vi "WS1050 16 DUT VSA-CV Sweep Ver1.1.vi"() -> ()   [LabVIEW 2012]
uses:
  Type Defs/WSVCAP SHL I2C DUT Mask Mode Enum.ctl
  <vilib>/Utility/file.llb/Read From Spreadsheet File (DBL).vi
  SubVI/Agilent E363X Series/Agilent E363X Series.lvlib
  SubVI/keithley_2000/Keithley 2000/Keithley 2000.lvlib
  SubVI/2012_Keithley 24XX/Keithley 24XX.lvlib
panel:
  out "Voltage Out":dbl[](array[numeric])
  out "C1 Out":dbl[][](array[numeric])
  out "VISA resource name out":refnum<visa-resource-name>="GPIB0::3::INSTR"
  out "date string":string="5/19/2014"
  out "PS1 Out":refnum<visa-resource-name>
  out "Ke2000 Out":refnum<visa-resource-name>="GPIB0::9::INSTR"
  in  "Tab Control":enum32{"Inst Control", "Data Output", "Graphs"}(tab)=enum."Data Output"
  out "AD7747 Values":string[][](table)
  in  "Lot#":string="WS1050"
  in  "Wafer#":string="T7-EB"
  in  "File Name":string="WS1050_T7_VSA_CV"
  in  "TMN DC\\CAP Data Log File Path":path=path "C:/WS1050 16 DUT Data"
  in  "SN":string[](array[string])=["1", "2", "3", "4", "5", "6", "7", "8", "9", "10", "11", "12", "13", "14", "15", "16"]
  in  "Test Program":string="WS1050 16 DUT VSA_CV Sweep Ver1.0"
  out "Current Date":string="8/28/2014"
  out "Current Time":string="0950"
  in  "Start Date":string="4/24/2014"
  in  "Start Time":string="1542"
  in  "Comment":string="5X0p5"
  in  "OK Button":bool
  in  "Calibration":bool
  in  "Control Setting":bool
  in  "CP Setting":i32(ring) items=["CP OFF", "CP ON", "CP 35V", "CP 40V", "DVA OFF", "DVA ON", "Reg1 ON", "Reg1 OFF", "Reg2 ON", "Reg2 OFF", "Reg3 ON", "Reg3 OFF"]
  in  "VDD(V)":dbl=3.3 format="%.3g"
  in  "SPI Clock Rate (Hz)":dbl=1000000.0 caption="Meas Speed" format="%.1p Hz"
  out "AR  Measurent(Hz)":dbl
  in  "PS1 Source":refnum<visa-resource-name>="GPIB0::5::INSTR"
  in  "Ke2000":refnum<visa-resource-name>="GPIB0::9::INSTR"
  out "Simulate FPGA":bool
  out "Online":bool
  in  "Ke2400":refnum<visa-resource-name>="GPIB0::3::INSTR"
  in  "Initialize AD7747":bool
  in  "DUT Mask Mode":T1=enum."All"
  in  "RFFE Slave Address":u8=7 caption="Slave Address" format="0x%02x"
  out "Activity Log":string="05/19/2014 -- 12:24:35.853::WSVCAP::APP::Application Started\n05/19/2014 -- 12:24:37.606::WSVCAP::WSVCAP SHL::WR I2C-REG:0x0A;MASK:0xFFFFFFFFFFFF;C1 DATA:22:22:22:22:22:22:22:22:22:22:22:22:22:22:22:22;C2 DATA:22:22:22:22:22:22:22:22:22:22:22:22:22:22:22:22;C3 DATA:22:22:22:22:22:22:22:22:22:22:22:22:22:22:22:22\r\n05/19/2014 -- 12:24:37.773::WSVCAP::WSVCAP SHL::WR I2C-ST:0,0,4,1\r\n05/19/2014 -- 12:24:37.903::WSVCAP::WSVCAP SHL::RD I2C-BYTES:4;ADD:0x00;MASK:0xFFFFFFFFFFFF\r\n05/19/2014 -- 12:24:38.045::WSVCAP::WSVCAP SHL::RD I2C:C1 DATA:2:2:2:2:2:2:2:2:2:2:2:2:2:2:2:2|A7:A9:AA:82:82:7F:82:81:82:81:83:82:81:82:82:81|46:36:BB:88:44:A3:E9:2B:32:20:ED:25:BB:3D:68:B|2C:6A:EB:A7:22:56:FE:CC:36:82:D7:B0:3B:48:F9:CC;C2 DATA:2:2:2:2:2:2:2:2:2:2:2:2:2:2:2:2|94:94:94:80:80:80:80:80:81:7E:7E:81:80:7E:80:80|47:33:15:82:62:B:E8:1C:D7:C3:7D:41:7C:B7:4C:2A|C4:B4:AE:8:1E:D1:4E:37:11:C0:6F:63:42:9D:63:B5;C3 DATA:2:2:2:2:2:2:2:2:2:2:2:2:2:2:2:2|95:95:95:81:81:7E:81:80:84:7D:80:83:81:7E:7F:80|AB:C4:14:B5:7B:52:DF:C9:79:5D:5F:30:99:31:1E:F4|6E:5C:F7:A8:C3:EB:7B:EF:33:92:89:77:4D:67:75:DD;STATUS:0:0:4:0\r\n05/19/2014 -- 12:24:38.046::WSVCAP::WSVCAP SHL::WR I2C-REG:0x0A;MASK:0xFFFFFFFFFFFF;C1 DATA:22:22:22:22:22:22:22:22:22:22:22:22:22:22:22:22;C2 DATA:22:22:22:22:22:22:22:22:22:22:22:22:22:22:22:22;C3 DATA:22:22:22:22:22:22:22:22:22:22:22:22:22:22:22:22\r\n05/19/2014 -- 12:24:38.089::WSVCAP::WSVCAP SHL::WR I2C-ST:0,0,4,1\r\n05/19/2014 -- 12:24:38.219::WSVCAP::WSVCAP SHL::RD I2C-BYTES:4;ADD:0x00;MASK:0xFFFFFFFFFFFF\r\n05/19/2014 -- 12:24:38.362::WSVCAP::WSVCAP SHL::RD I2C:C1 DATA:2:2:2:2:2:2:2:2:2:2:2:2:2:2:2:2|A7:AB:AA:82:82:82:83:83:82:82:82:82:7F:82:82:81|4B:32:96:83:3E:61:43:17:25:62:AB:4D:A2:40:2E:5|3C:76:2B:B4:EE:E4:A9:1A:AA:A:26:C7:21:2E:87:5B;C2 DATA:2:2:2:2:2:2:2:2:2:2:2:2:2:2:2:2|94:94:94:80:80:80:80:80:80:7F:80:81:80:80:7F:80|4A:32:19:7D:19:6C:79:46:61:7F:4B:B8:A5:30:F3:14|B4:70:A:8C:9C:DC:43:FA:1E:A:C6:21:A:A9:13:F3;C3 DATA:2:2:2:2:2:2:2:2:2:2:2:2:2:2:2:2|95:97:94:81:80:81:82:81:80:7E:81:84:7F:81:80:80|B2:32:D0:A7:9E:4C:AB:D4:EE:D9:F0:82:B7:91:7:FF|C1:91:B6:3D:D8:E:1B:4F:9F:6A:F1:6C:E7:3F:7:BA;STATUS:0:0:4:0\r\n05/19/2014 -- 12:24:38.364::WSVCAP::WSVCAP SHL::WR I2C-REG:0x0A;MASK:0xFFFFFFFFFFFF;C1 DATA:22:22:22:22:22:22:22:22:22:22:22:22:22:22:22:22;C2 DATA:22:22:22:22:22:22:22:22:22:22:22:22:22:22:22:22;C3 DATA:22:22:22:22:22:22:22:22:22:22:22:22:22:22:22:22\r\n05/19/2014 -- 12:24:38.406::WSVCAP::WSVCAP SHL::WR I2C-ST:0,0,4,1\r\n05/19/2014 -- 12:24:38.536::WSVCAP::WSVCAP SHL::RD I2C-BYTES:4;ADD:0x00;MASK:0xFFFFFFFFFFFF\r\n05/19/2014 -- 12:24:38.678::WSVCAP::WSVCAP SHL::RD I2C:C1 DATA:2:2:2:2:2:2:2:2:2:2:2:2:2:2:2:2|A7:A9:AB:82:82:81:82:82:82:82:82:82:82:82:82:81|46:71:4C:87:43:3D:7F:FC:25:4F:8E:54:97:3E:60:8C|AA:F4:1F:B5:CE:43:1F:36:9:87:9C:78:86:5:B6:8E;C2 DATA:2:2:2:2:2:2:2:2:2:2:2:2:2:2:2:2|94:94:94:80:7F:7F:80:80:80:80:80:81:80:80:80:80|49:36:18:7D:6E:C5:E4:3C:81:2E:41:D3:75:71:E3:72|E8:D3:E6:D1:E0:48:AE:D4:54:D:E8:8E:B4:41:68:4;C3 DATA:2:2:2:2:2:2:2:2:2:2:2:2:2:2:2:2|95:95:95:81:7F:7F:81:81:81:81:81:84:81:81:82:81|B3:F5:90:AB:82:69:7B:93:D0:77:E8:D5:E8:8C:84:E8|B9:AC:EE:2B:B6:71:8F:4A:74:31:56:BB:8A:B7:A0:C8;STATUS:0:0:4:0\r\n05/19/2014 -- 12:24:38.681::WSVCAP::WSVCAP SHL::WR I2C-REG:0x0A;MASK:0xFFFFFFFFFFFF;C1 DATA:22:22:22:22:22:22:22:22:22:22:22:22:22:22:22:22;C2 DATA:22:22:22:22:22:22:22:22:22:22:22:22:22:22:22:22;C3 DATA:22:22:22:22:22:22:22:22:22:22:22:22:22:22:22:22\r\n05/19/2014 -- 12:24:38.723::WSVCAP::WSVCAP SHL::WR I2C-ST:0,0,4,1\r\n05/19/2014 -- 12:24:38.854::WSVCAP::WSVCAP SHL::RD I2C-BYTES:4;ADD:0x00;MASK:0xFFFFFFFFFFFF\r\n05/19/2014 -- 12:24:38.996::WSVCAP::WSVCAP SHL::RD I2C:C1 DATA:2:2:2:2:2:2:2:2:2:2:2:2:2:2:2:2|A7:A9:AA:82:82:7F:83:81:82:81:84:82:7F:82:7F:82|43:FB:E:7F:3C:AD:35:35:26:A2:6C:21:4B:3D:8:6|63:9A:E1:F3:95:32:91:42:90:3C:78:1F:5C:D7:5F:D8;C2 DATA:2:2:2:2:2:2:2:2:2:2:2:2:2:2:2:2|94:94:94:80:80:80:80:80:81:80:7E:81:80:7E:7F:80|48:36:18:7F:5E:3D:69:83:DE:AE:A1:9E:31:AE:BB:96|15:A0:44:17:13:FD:CC:C8:6D:B2:EF:A7:C:C7:3B:F;C3 DATA:2:2:2:2:2:2:2:2:2:2:2:2:2:2:2:2|95:96:94:81:81:7E:82:80:84:80:80:84:7F:7E:7D:82|AD:3B:6D:A9:7C:57:9D:F5:7A:96:23:5C:36:2D:ED:5A|CD:46:DB:3B:C7:BD:70:60:33:B8:B:F7:63:A:51:4D;STATUS:0:0:4:0\r\n05/19/2014 -- 12:24:38.998::WSVCAP::WSVCAP SHL::WR I2C-REG:0x0A;MASK:0xFFFFFFFFFFFF;C1 DATA:22:22:22:22:22:22:22:22:22:22:22:22:22:22:22:22;C2 DATA:22:22:22:22:22:22:22:22:22:22:22:22:22:22:22:22;C3 DATA:22:22:22:22:22:22:22:22:22:22:22:22:22:22:22:22\r\n05/19/2014 -- 12:24:39.040::WSVCAP::WSVCAP SHL::WR I2C-ST:0,0,4,1\r\n05/19/2014 -- 12:24:39.170::WSVCAP::WSVCAP SHL::RD I2C-BYTES:4;ADD:0x00;MASK:0xFFFFFFFFFFFF\r\n05/19/2014 -- 12:24:39.311::WSVCAP::WSVCAP SHL::RD I2C:C1 DATA:2:2:2:2:2:2:2:2:2:2:2:2:2:2:2:2|A7:AA:AB:82:82:81:82:81:82:81:82:82:82:82:7F:82|44:F1:90:87:45:44:C8:2C:2C:F1:FC:1B:94:3B:3C:75|4A:49:95:19:99:73:64:3:23:24:F3:A2:5E:7F:C4:B6;C2 DATA:2:2:2:2:2:2:2:2:2:2:2:2:2:2:2:2|94:94:94:80:80:80:80:7F:80:80:7E:80:80:7E:7F:80|4C:36:17:7D:A8:9F:DE:C7:53:6D:8A:F4:41:A5:C6:E0|90:2E:24:C:D9:22:E4:76:3B:40:1D:53:33:B1:3E:4D;C3 DATA:2:2:2:2:2:2:2:2:2:2:2:2:2:2:2:2|95:97:95:81:81:7F:81:80:80:81:7F:82:81:7E:7D:82|AE:2B:A7:AB:CC:CD:A4:38:FD:17:80:F2:92:2D:45:C4|76:E5:D:B9:AD:B5:BA:8D:28:32:9E:42:B7:20:4A:D9;STATUS:0:0:4:0\r\n05/19/2014 -- 12:24:39.313::WSVCAP::WSVCAP SHL::WR I2C-REG:0x0A;MASK:0xFFFFFFFFFFFF;C1 DATA:22:22:22:22:22:22:22:22:22:22:22:22:22:22:22:22;C2 DATA:22:22:22:22:22:22:22:22:22:22:22:22:22:22:22:22;C3 DATA:22:22:22:22:22:22:22:22:22:22:22:22:22:22:22:22\r\n05/19/2014 -- 12:24:39.355::WSVCAP::WSVCAP SHL::WR I2C-ST:0,0,4,1\r\n05/19/2014 -- 12:24:39.486::WSVCAP::WSVCAP SHL::RD I2C-BYTES:4;ADD:0x00;MASK:0xFFFFFFFFFFFF\r\n05/19/2014 -- 12:24:39.628::WSVCAP::WSVCAP SHL::RD I2C:C1 DATA:2:2:2:2:2:2:2:2:2:2:2:2:2:2:2:2|A7:A9:AA:82:82:82:83:82:82:82:82:82:7F:82:7F:82|47:18:E4:87:3E:E7:6:65:25:92:37:38:A8:3E:89:85|7C:A7:7:2B:A3:7A:EC:EF:89:ED:F4:D3:D8:BC:3A:F5;C2 DATA:2:2:2:2:2:2:2:2:2:2:2:2:2:2:2:2|94:94:94:80:7F:80:80:7F:81:80:7E:80:80:80:81:80|49:37:17:80:76:25:6A:F8:DF:55:97:4D:B8:5B:2B:B1|13:E3:9A:3E:1A:2D:4F:B6:DB:E9:61:FA:8B:D6:9:CC;C3 DATA:2:2:2:2:2:2:2:2:2:2:2:2:2:2:2:2|95:95:95:81:7F:80:82:81:84:80:7F:81:80:81:7F:82|AF:93:3B:AF:5B:11:82:E4:7E:C3:2D:72:9:96:D9:A|DB:96:F2:10:5F:64:9A:C6:98:12:27:7D:10:D3:20:D9;STATUS:0:0:4:0\r\n05/19/2014 -- 12:24:40.132::WSVCAP::WSVCAP SHL::CLOSE\r\n"
  in  "C1 Cap DAC":u8=128 caption="B Data In" format="0x%02x"
  in  "C2 Cap DAC":u8=128 caption="B Data In" format="0x%02x"
  in  "C3 Cap DAC":u8=128 caption="B Data In" format="0x%02x"
  out "IDD Brd(uA)":string
  in  "VSA_IDD(A)":dbl=0.1
  out "Previous Time":string="12:20:26 PM"
  out "STATUS":string="Idle...."
  in  "stop":bool
  out "VSA_C1_T0":string[](array[string])
  out "VSA_Value(pF)":string[][](array[string])
  out "VSA_C3_T0":string[](array[string])
  out "VSA_C2_T0":string[](array[string])
  in  "VSA Voltag Path":path=path "C:/VSA Voltage Sweep/VSA_Voltage_Seq_0-10-24V Step2V.txt"
  in  "VSA_CV Voltage Path":path=path "C:/VSA Voltage Sweep/VSA_Voltage_Seq_0-10-24V Step2V.txt"
  out "CP Current(uA)":string[](array[string])
  in  "Abort":bool
  out "Running Loops":i32=1
  in  "VSA_CV Reg Setting":i32(ring) items=["Reg1 ON", "Reg1 OFF", "Reg2 ON", "Reg2 OFF", "Reg3 ON", "Reg3 OFF", "All ON", "All OFF"]
  in  "VSA Test":bool=TRUE
  in  "error in (no error)":errorcluster
  out "error out":errorcluster
  out "error out 2":errorcluster
  out "Bank 3 Graph":cluster{"Y":dbl[], "Y":dbl[]}[](graph)
  out "Bank 2 Graph":cluster{"Y":dbl[], "Y":dbl[]}[](graph)
  out "Bank 1 Graph":cluster{"Y":dbl[], "Y":dbl[]}[](graph)
  out "C2 Plot":dbl[][](graph)
  out "C1 Plot":dbl[][](graph)
  out "C3 Plot":dbl[][](graph)
  # "Company:  WiSpry Inc 20 Fairbanks \nSte 198 Irvine CA 92618\n\nAuthor:  Andy V Tran\nCreated:  09/16/2015\nLabVIEW 2012 Pro\nTP:  WS1050 16 DUT VSA_CV Ver1.1\nFPGA Version: WS_VCAP Driver 024"
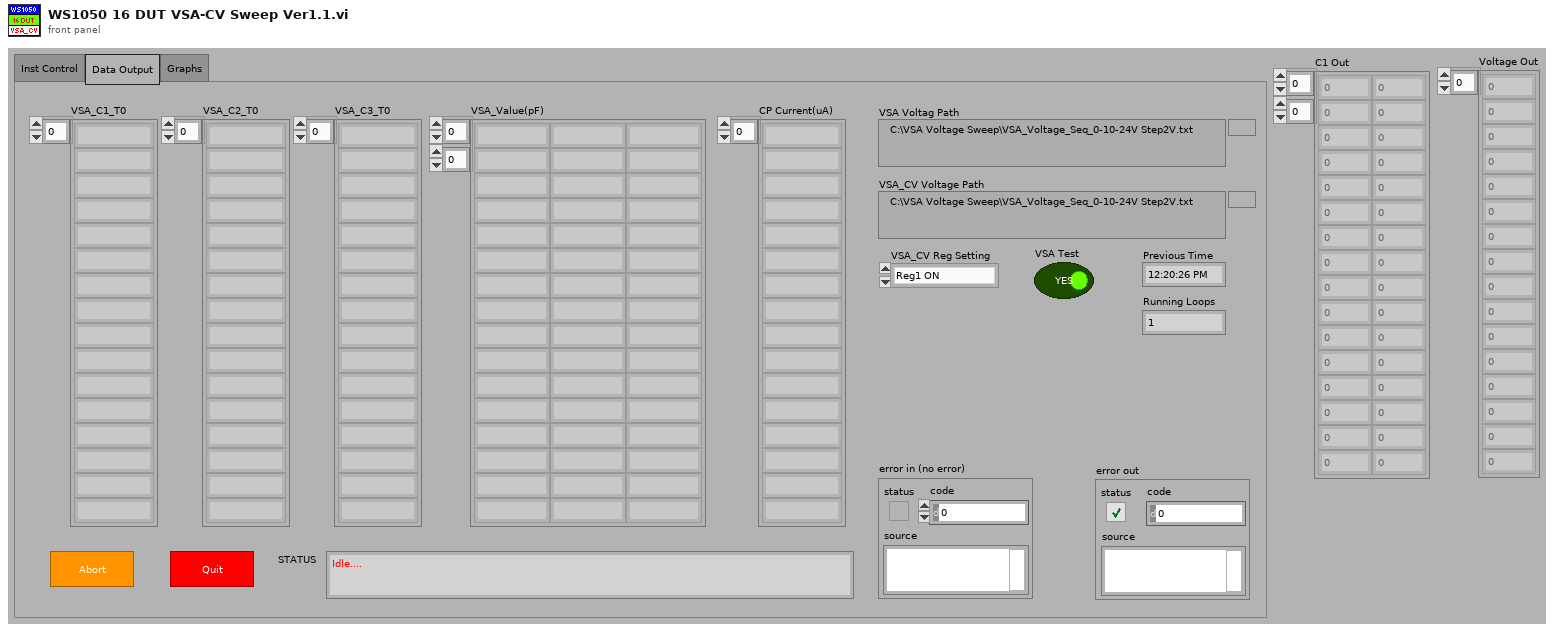
[diagram p1: front panel]
types:
  T1 = typedef "WSVCAP SHL I2C DUT Mask Mode Enum.ctl" = enum16{"Custom", "C1", "C2", "C3", "All"}
  T2 = typedef "WSVCAP SHL Core System Cluster.ctl" = cluster{"Settings":T3, "FPGA Resource":tag, "Online":bool, "I2C Wait Ticks":u32, "SPI Wait Ticks":u32, "RFFE Wait Ticks":u32}
  T3 = typedef "WSVCAP SHL I2C Settings Cluster.ctl" = cluster{"FPGA Resource Name":string, "I2C Slave Address":u8, "I2C Clock Rate (Hz)":dbl, "SPI Clock Rate (Hz)":dbl, "RFFE Slave Address":u8, "RFFE Clock Rate (Hz)":dbl, "Simulate FPGA":bool, "C1 Cap DAC Default":u8, "C2 Cap DAC Default":u8, "C3 Cap DAC Default":u8}
  T4 = enum16{"Idle...", "Voltage 1", "Voltage 2", "Voltage 3"}[]
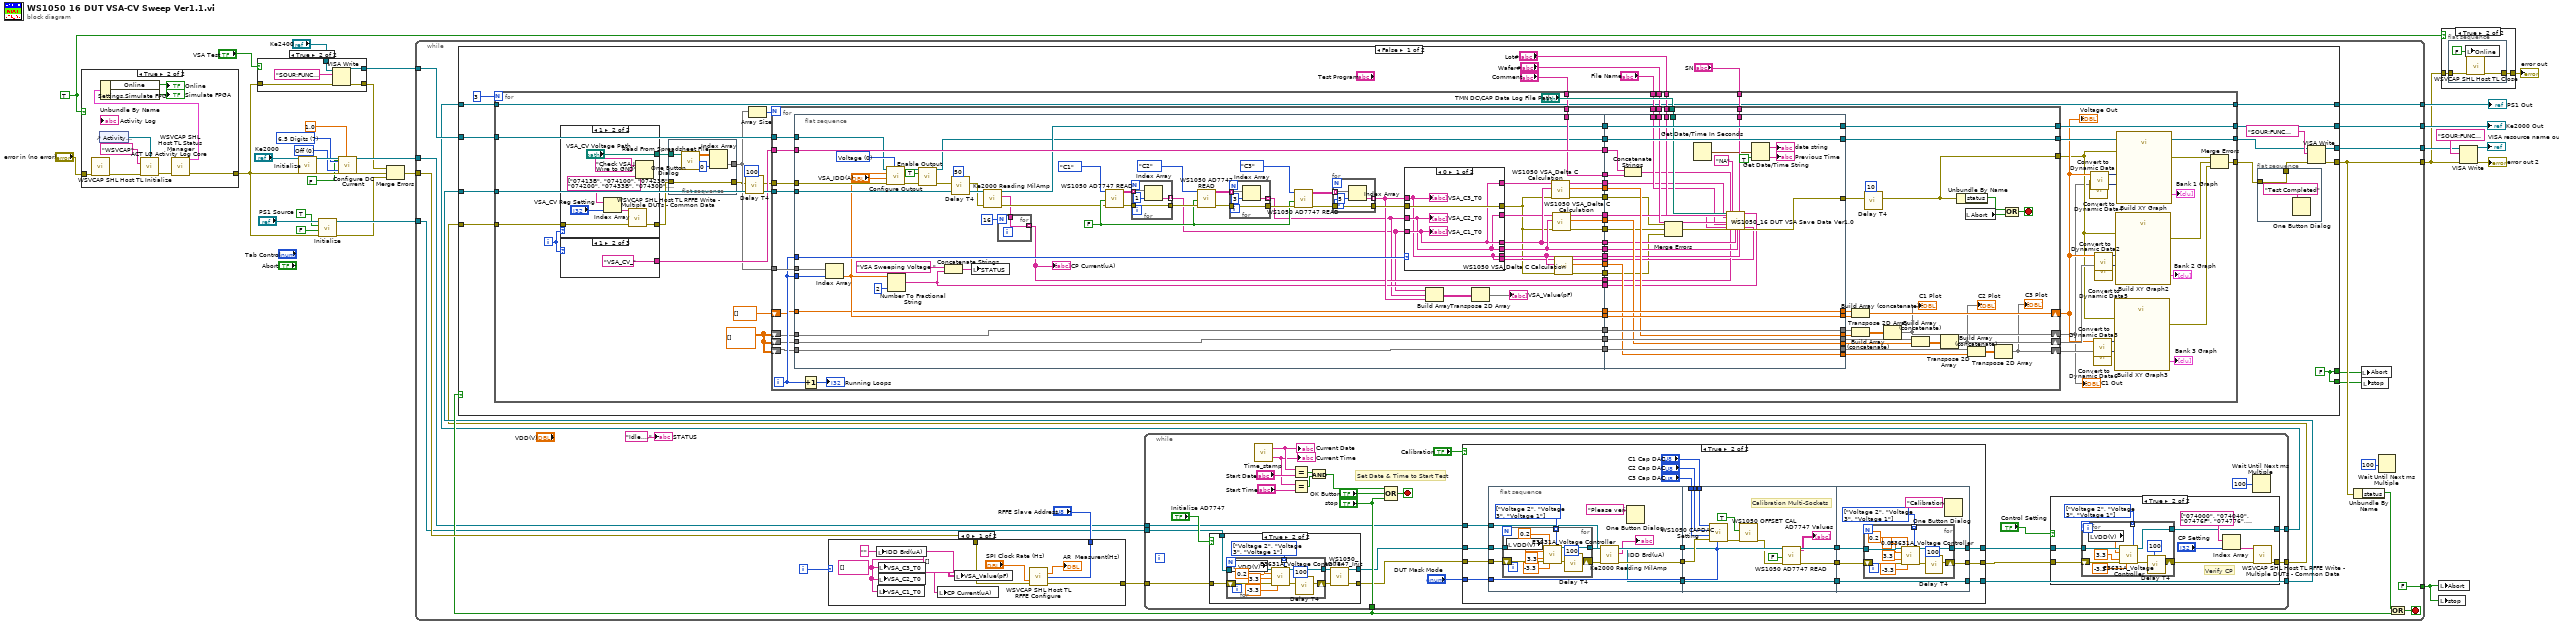
[diagram p0: block diagram]
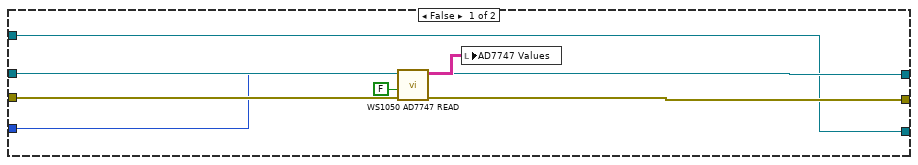
[diagram p8: hidden frame]
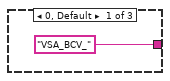
[diagram p9: hidden frame]
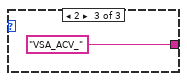
[diagram p10: hidden frame]
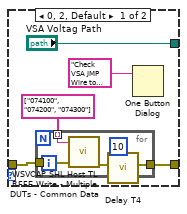
[diagram p11: hidden frame]
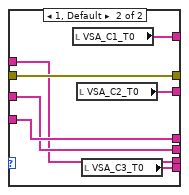
[diagram p12: hidden frame]
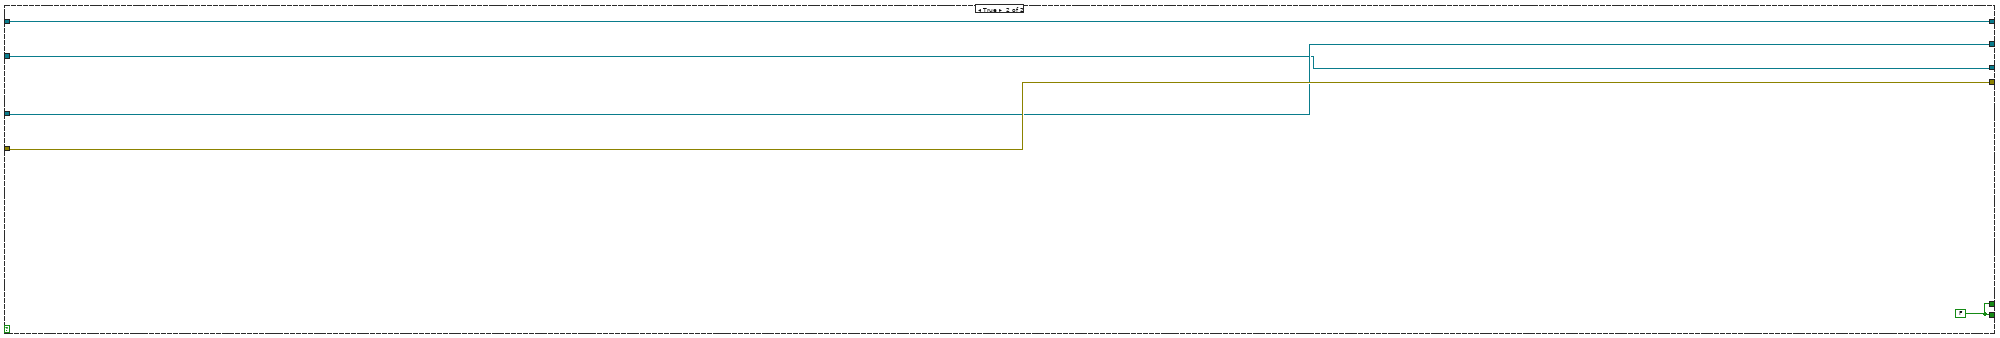
[diagram p13: hidden frame]
diagram:
  w17 = TRUE
  w23 = u16 0 items=["Off", "Moving Filter", "Repeating Filter"] ("Digital Filter (0: Off)")
  w24 = u16 7 items=["3.5 Digits"=4, "4.5 Digits"=5, "5.5 Digits"=6, "6.5 Digits"=7] ("Resolution (7: 6.5 digits)")
  n1 = case shown="True" w17 {
    tunnel: "error in (no error)" -> [w32 w33]
    tunnel: [w32 w40] -> w5
    frame False {
    }
    frame True {
      n2 = call "WSVCAP SHL Host TL Initialize.vi"("error in"=w33) -> ("error out"=w34:errorcluster)  [unwired: 13 in, 1 out]
      n3 = control-ref of="Activity Log"() -> (w36:refnum<vi>)
      n4 = call "ACT LG Activity Log Core.vi"("Display Ref"=w36, "Source"="WSVCAP", "Error In (no error)"=w34) -> ("Error Out"=w35:errorcluster)  [unwired: 11 in, 1 out]
      n5 = call "WSVCAP SHL Host TL Status Manager.vi"("error in"=w35) -> ("System Out"=w41:T2, "error out"=w40:errorcluster)  [unwired: 13 in]
      n6 = Unbundle By Name(w41) -> ("Online"=→"Online":bool, "Settings.Simulate FPGA"=→"Simulate FPGA":bool)
    }
  }
  n7 = case shown="True" "VSA Test" {
    tunnel: w5 -> [w42 w47]
    tunnel: [w43 w46] -> w14
    tunnel: [w42 w45] -> w9
    tunnel: "Ke2400" -> [w43 w44]
    frame False {
    }
    frame True {
      n8 = VISA Write(VISA resource name=w44, write buffer="SOUR:FUNC VOLT;VOLT:MODE FIX;RANG 100;LEV 0.0;:SENS:FUNC \"CURR\";CURR:PROT 60E-3;RANG 100E-3;:OUTP ON", error in (no error)=w47) -> (VISA resource name out=w46:refnum<visa-resource-name>, error out=w45:errorcluster)  [unwired: 1 out]
    }
  }
  n9 = call "Initialize.vi"("VISA resource name"="Ke2000", "error in (no error)"=w5) -> ("VISA resource name out"=w26:refnum<visa-resource-name>, "error out"=w25:errorcluster)  [unwired: 16 in]
  n10 = call "Initialize.vi"("error in (no error)"=w5, "Reset? (T: Yes)"=FALSE, "ID Query? (T: Yes)"=TRUE, "VISA resource name"="PS1 Source") -> ("error out"=w4:errorcluster, "VISA resource name out"=w29:refnum<visa-resource-name>)  [unwired: 6 in]
  n11 = call "Configure DC Current.vi"("VISA resource name"=w26, "Resolution (7: 6.5 digits)"=w24, "error in (no error)"=w25, "Auto Range? (T: Auto)"=FALSE, "Digital Filter (0: Off)"=w23, "Custom Range (0 A)"=1.0) -> ("VISA resource name out"=w21:refnum<visa-resource-name>, "error out"=w6:errorcluster)  [unwired: 12 in]
  n12 = Merge Errors(w9, w6, w4) -> (w15:errorcluster)
  n13 = while {
    tunnel: w15 -> [w63]
    tunnel: [w52] -> w11
    tunnel: w29 -> [w56]
    tunnel: w21 -> [w57]
    tunnel: [w66] -> w20
    tunnel: [w65] -> w19
    tunnel: w14 -> [w62]
    tunnel: [w61] -> w12
    tunnel: [FALSE] -> w3
    i -> [w64]
    stop <- w68 stop-if-true
    n14 = case shown="0" w64 {
      tunnel: w63 -> [w78 w79]
      tunnel: [w77 w79] -> w59
      tunnel: "RFFE Slave Address" -> [w75 _]
      frame 0 {
        w72 = string[] []
        n15 = local write "IDD Brd(uA)"("" ("uA")) -> ()
        n16 = local write "VSA_C1_T0"(w72) -> ()
        n17 = local write "VSA_C3_T0"(w72) -> ()
        n18 = local write "VSA_C2_T0"(w72) -> ()
        n19 = local write "CP Current(uA)"(w72) -> ()
        n20 = local write "VSA_Value(pF)"(string[][] []) -> ()
        n21 = call "WSVCAP SHL Host TL RFFE Configure.vi"("RFFE Slave Address"=w75, "Clock Rate (Hz)"="SPI Clock Rate (Hz)", "error in"=w78) -> ("Actual Rate (Hz)"=→"AR  Measurent(Hz)":dbl, "error out"=w77:errorcluster)  [unwired: 11 in]
      }
      frame 1, Default {
      }
    }
    n22 = while {
      tunnel: ["stop"] -> w60
      tunnel: w59 -> [w90]
      tunnel: [w81] -> w53
      tunnel: w56 -> [w88]
      tunnel: w57 -> [w83]
      tunnel: [w84] -> w55
      tunnel: [w82] -> w54
      stop <- w97 stop-if-true
      # "Set Date & Time to Start Test"
      n23 = case shown="True" "Initialize AD7747" {
        tunnel: w90 -> [w106 w111]
        tunnel: [w106 w107] -> w89
        tunnel: w88 -> [w105 w109]
        tunnel: [w105 w108] -> w87
        frame False {
        }
        frame True {
          w112 = T4 [enum."Voltage 2", enum."Voltage 3", enum."Voltage 1"] items=["Idle...", "Voltage 1", "Voltage 2", "Voltage 3"]
          n24 = for {
            tunnel: w109 -> [w122]
            tunnel: w112 -> [w119] mode=indexing
            tunnel: [w118] -> w108
            shift-right: [w114] -> w110
            shift-left: w111 -> [w123]
            n25 = local read "VDD(V)"() -> (w117:dbl)
            n26 = call "E3631A_Voltage Controller.vi"("VISA resource name"=w122, "I_VDD(A)"=0.2, "Channel Controller"=w119, "Voltage 1"=w117, "Voltage 2"=3.3, "error in (no error)"=w123, "Voltage 3"=-3.3) -> ("VISA resource name out"=w118:refnum<visa-resource-name>, "error out"=w113:errorcluster)  [unwired: 7 in]
            n27 = call "Delay T4.vi"("milliseconds to wait"=u32 100, "error in (no error)"=w113) -> ("error out"=w114:errorcluster)  [unwired: 9 in]
          }
          n28 = call "WS1050_AD7747_Init.vi"("error in"=w110) -> ("error out"=w107:errorcluster)  [unwired: 10 in]
        }
      }
      n29 = call "Time_stamp.vi"() -> ("date/time string"=w102:string, "date string"=w104:string)  [unwired: 2 in]
      "Current Date" <- w104
      "Current Time" <- w102
      n30 = Equal?(x=w104, y="Start Date") -> (x = y?=w100:bool)
      n31 = Equal?(x=w102, y="Start Time") -> (x = y?=w99:bool)
      n32 = And(x=w100, y=w99) -> (x .and. y?=w96:bool)
      n33 = Compound Arithmetic op=OR(w96, "OK Button", "stop") -> (w97:bool)
      n34 = case shown="True" "Calibration" {
        tunnel: w89 -> [w150 w168]
        tunnel: [w149 w165] -> w80
        tunnel: w87 -> [w148 w164]
        tunnel: "DUT Mask Mode" -> [w147 w160]
        tunnel: [w148 w159] -> w85
        tunnel: w83 -> [w146 w155]
        tunnel: [w146 w152] -> w82
        frame False {
          n35 = call "WS1050 AD7747 READ.vi"("error in"=w150, "Log (T)"=FALSE, "DUT Mask Mode (All)"=w147) -> ("error out"=w149:errorcluster, "AD7747 Values"=w151:string[][])  [unwired: 7 in]
          n36 = local write "AD7747 Values"(w151) -> ()
        }
        frame True {
          n37 = flat-sequence {
            tunnel: w168 -> [w177]
            tunnel: [w172] -> w167
            tunnel: w164 -> [w176]
            tunnel: [w175] -> w163
            tunnel: w160 -> [w174]
            tunnel: [w174] -> w161
            tunnel: w155 -> [w170]
            tunnel: [w169] -> w154
            tunnel: w167 -> [w203]
            tunnel: [w202] -> w166
            tunnel: w163 -> [w201]
            tunnel: [w201] -> w162
            tunnel: w161 -> [w200]
            tunnel: "C1 Cap DAC" -> [w196]
            tunnel: "C2 Cap DAC" -> [w195]
            tunnel: "C3 Cap DAC" -> [w194]
            tunnel: w154 -> [w193]
            tunnel: [w193] -> w153
            tunnel: w166 -> [w206]
            tunnel: [w209] -> w165
            tunnel: w162 -> [w208]
            tunnel: [w205] -> w159
            tunnel: w153 -> [w204]
            tunnel: [w204] -> w152
            frame #0 {
              w178 = T4 [enum."Voltage 2", enum."Voltage 3", enum."Voltage 1"] items=["Idle...", "Voltage 1", "Voltage 2", "Voltage 3"]
              n38 = for {
                tunnel: w176 -> [w189]
                tunnel: w178 -> [w186] mode=indexing
                tunnel: [w185] -> w175
                shift-right: [w183] -> w171
                shift-left: w177 -> [w190]
                n39 = local read "VDD(V)"() -> (w180:dbl)
                n40 = call "E3631A_Voltage Controller.vi"("VISA resource name"=w189, "I_VDD(A)"=0.2, "Channel Controller"=w186, "Voltage 1"=w180, "Voltage 2"=3.3, "error in (no error)"=w190, "Voltage 3"=-3.3) -> ("VISA resource name out"=w185:refnum<visa-resource-name>, "error out"=w182:errorcluster)  [unwired: 7 in]
                n41 = call "Delay T4.vi"("milliseconds to wait"=u32 100, "error in (no error)"=w182) -> ("error out"=w183:errorcluster)  [unwired: 9 in]
              }
              n42 = call "Ke2000 Reading MilAmp.vi"("error in (no error)"=w171, "VISA resource name"=w170) -> ("error out"=w172:errorcluster, "uA"=→"IDD Brd(uA)":string, "VISA resource name out"=w169:refnum<visa-resource-name>)  [unwired: 7 in]
              n43 = One Button Dialog(message="Please verify all sockets should be empty...") -> ()  [unwired: 1 in, 1 out]
            }
            frame #1 {
              # "Calibration Multi-Sockets"
              n44 = call "WS1050 CAPDAC Setting.vi"("DUT Mask Mode (All)"=w200, "error in"=w203, "C3 Cap DAC"=w194, "C2 Cap DAC"=w195, "C1 Cap DAC"=w196) -> ("error out"=w198:errorcluster)  [unwired: 5 in, 1 out]
              n45 = call "WS1050 OFFSET CAL.vi"("error in"=w198, "OFFSET CAL"=TRUE ("Read?")) -> ("error out"=w197:errorcluster)  [unwired: 8 in, 1 out]
              n46 = call "WS1050 AD7747 READ.vi"("error in"=w197, "Log (T)"=FALSE, "DUT Mask Mode (All)"=w200) -> ("error out"=w202:errorcluster, "AD7747 Values"=→"AD7747 Values":string[][])  [unwired: 7 in]
            }
            frame #2 {
              w207 = T4 [enum."Voltage 2", enum."Voltage 3", enum."Voltage 1"] items=["Idle...", "Voltage 1", "Voltage 2", "Voltage 3"]
              n47 = for {
                tunnel: w208 -> [w221]
                tunnel: w207 -> [w217] mode=indexing
                tunnel: [w216] -> w205
                shift-right: [w212] -> w209
                shift-left: w206 -> [w218]
                n48 = call "E3631A_Voltage Controller.vi"("VISA resource name"=w221, "I_VDD(A)"=0.2, "Channel Controller"=w217, "Voltage 1"=0.0, "Voltage 2"=3.3, "error in (no error)"=w218, "Voltage 3"=-3.3) -> ("VISA resource name out"=w216:refnum<visa-resource-name>, "error out"=w211:errorcluster)  [unwired: 7 in]
                n49 = call "Delay T4.vi"("milliseconds to wait"=u32 100, "error in (no error)"=w211) -> ("error out"=w212:errorcluster)  [unwired: 9 in]
              }
              n50 = One Button Dialog(message="Calibration Completed....") -> ()  [unwired: 1 in, 1 out]
            }
          }
        }
      }
      n51 = case shown="True" "Control Setting" {
        tunnel: [w124 w127] -> w81
        tunnel: w85 -> [w125 w130]
        tunnel: [w125 w128] -> w84
        tunnel: w80 -> [w124 w126]
        frame False {
        }
        frame True {
          w131 = T4 [enum."Voltage 2", enum."Voltage 3", enum."Voltage 1"] items=["Idle...", "Voltage 1", "Voltage 2", "Voltage 3"]
          # "Verify CP"
          n52 = for {
            tunnel: w130 -> [w143]
            tunnel: w131 -> [w140] mode=indexing
            shift-right: [w137] -> w129
            shift-left: w126 -> [w144]
            tunnel: [w135] -> w128
            n53 = local read "VDD(V)"() -> (w139:dbl)
            n54 = call "E3631A_Voltage Controller.vi"("VISA resource name"=w143, "Channel Controller"=w140, "Voltage 1"=w139, "Voltage 2"=3.3, "error in (no error)"=w144, "Voltage 3"=-3.3) -> ("VISA resource name out"=w135:refnum<visa-resource-name>, "error out"=w138:errorcluster)  [unwired: 8 in]
            n55 = call "Delay T4.vi"("milliseconds to wait"=u32 100, "error in (no error)"=w138) -> ("error out"=w137:errorcluster)  [unwired: 9 in]
          }
          n56 = Index Array(array=string[] ["074000", "074040", "07476F", "074776", "074820", "074800", "07413B", "074100", "07423B", "074200", "07433B", "074300"], index="CP Setting") -> (element=w132:string)
          n57 = call "WSVCAP SHL Host TL RFFE Write - Multiple DUTs - Common Data.vi"("Data Out"=w132, "error in"=w129) -> ("error out"=w127:errorcluster)  [unwired: 13 in]
        }
      }
      n58 = Wait Until Next ms Multiple(millisecond multiple=u32 100) -> ()  [unwired: 1 out]
    }
    n59 = case shown="False" w60 {
      tunnel: w53 -> [w237 w501]
      tunnel: [w226 w501] -> w52
      tunnel: w55 -> [w230 w499]
      tunnel: w54 -> [w238 w500]
      tunnel: [w229 w500] -> w66
      tunnel: [w227 w499] -> w65
      tunnel: w62 -> [w240 w498]
      tunnel: [w236 w498] -> w61
      tunnel: [w228 w497] -> w50
      tunnel: [w228 w497] -> w49
      frame False {
        w228 = FALSE
        n60 = for {
          N: 3 -> [_]
          tunnel: w240 -> [w282]
          tunnel: w238 -> [w281]
          tunnel: w237 -> [w278]
          tunnel: [w280] -> w225
          tunnel: [w250] -> w224
          tunnel: "Comment" -> [w276]
          tunnel: "Lot#" -> [w275]
          tunnel: "Wafer#" -> [w274]
          tunnel: "SN" -> [w273]
          tunnel: "File Name" -> [w272]
          tunnel: [w270] -> w227
          tunnel: w230 -> [w270]
          tunnel: [w269] -> w229
          i -> [w277]
          w254 = dbl[][] []
          n61 = case shown="1" w277 {
            tunnel: ["VSA Voltag Path" "VSA_CV Voltage Path"] -> w256
            tunnel: w278 -> [w293 w303]
            tunnel: [w294 w302] -> w257
            frame 0, 2, Default {
              n62 = for {
                tunnel: [w300] -> w294
                tunnel: w293 -> [w299]
                tunnel: string[] ["074100", "074200", "074300"] -> [w298] mode=indexing
                n63 = call "WSVCAP SHL Host TL RFFE Write - Multiple DUTs - Common Data.vi"("Data Out"=w298, "error in"=w299) -> ("error out"=w301:errorcluster)  [unwired: 13 in]
                n64 = call "Delay T4.vi"("milliseconds to wait"=u32 10, "error in (no error)"=w301) -> ("error out"=w300:errorcluster)  [unwired: 9 in]
              }
              n65 = One Button Dialog(message="Check VSA JMP Wire to SRC") -> ()  [unwired: 1 in, 1 out]
            }
            frame 1 {
              n66 = Index Array(array=string[] ["07413B", "074100", "07423B", "074200", "07433B", "074300", "0702013B3B3B", "070201000000"], index="VSA_CV Reg Setting") -> (element=w304:string)
              n67 = call "WSVCAP SHL Host TL RFFE Write - Multiple DUTs - Common Data.vi"("Data Out"=w304, "error in"=w303) -> ("error out"=w302:errorcluster)  [unwired: 13 in]
              n68 = One Button Dialog(message="Check VSA JMP Wire to GND") -> ()  [unwired: 1 in, 1 out]
            }
          }
          n69 = case shown="1" w277 {
            tunnel: ["VSA_BCV_" "VSA_CV_" "VSA_ACV_"] -> w271
            frame 0, Default {
            }
            frame 1 {
            }
            frame 2 {
            }
          }
          n70 = flat-sequence {
            tunnel: w257 -> [w288]
            tunnel: [w288] -> w246
            tunnel: w256 -> [w287]
            tunnel: [w285] -> w255
            frame #0 {
              n71 = call-poly <vilib>:"Read From Spreadsheet File.vi"("file path (dialog if empty)"=w287) -> ("all rows"=w284:dbl[][])  [unwired: 6 in, 4 out]
              n72 = Index Array(array=w284, index (col)=0 ("disabled index (col)")) -> (element=w285:dbl[])  [unwired: 1 in]
            }
          }
          n73 = call "Delay T4.vi"("milliseconds to wait"=u32 100, "error in (no error)"=w246) -> ("error out"=w245:errorcluster)  [unwired: 9 in]
          n74 = Array Size(array=w255) -> (size(s)=w279:i32)
          n75 = for {
            N: w279 -> [_]
            tunnel: w255 -> [w371]
            tunnel: w281 -> [w370]
            tunnel: "TMN DC\\CAP Data Log File Path" -> [w358]
            tunnel: w282 -> [w312]
            tunnel: [w368] -> w251
            tunnel: w245 -> [w366]
            tunnel: [w362] -> w280
            tunnel: w276 -> [w344]
            tunnel: w275 -> [w351]
            tunnel: w274 -> [w350]
            tunnel: w273 -> [w349]
            tunnel: w272 -> [w348]
            tunnel: w271 -> [w347]
            tunnel: [w342] -> w269
            shift-right: [w337] -> w252
            shift-left: dbl[] [] -> [w336]
            shift-right: [w317] -> w243
            shift-left: w254 -> [w332]
            shift-right: [w315] -> w261
            shift-left: w254 -> [w330]
            shift-right: [w313] -> w259
            shift-left: w254 -> [w329]
            i -> [w357]
            stop <- w367 stop-if-true
            n76 = flat-sequence {
              tunnel: w371 -> [w435]
              tunnel: w370 -> [w411]
              tunnel: w357 -> [w434]
              tunnel: w366 -> [w436]
              tunnel: [w380] -> w363
              tunnel: [w404] -> w361
              tunnel: [w405] -> w360
              tunnel: [w406] -> w359
              tunnel: w357 -> [w413]
              tunnel: [w399] -> w356
              tunnel: [w407] -> w355
              tunnel: [w403] -> w354
              tunnel: [w402] -> w353
              tunnel: [w401] -> w352
              tunnel: w347 -> [w397]
              tunnel: [w397] -> w346
              tunnel: [w396] -> w345
              tunnel: w344 -> [w396]
              tunnel: [w395] -> w343
              tunnel: [w394] -> w339
              tunnel: w336 -> [w393]
              tunnel: [w393] -> w335
              tunnel: [w388] -> w333
              tunnel: w332 -> [w388]
              tunnel: [w389] -> w331
              tunnel: w330 -> [w389]
              tunnel: w329 -> [w392]
              tunnel: [w392] -> w328
              tunnel: [w391] -> w327
              tunnel: [w390] -> w326
              tunnel: [w387] -> w325
              tunnel: w312 -> [w381]
              tunnel: [w374] -> w311
              tunnel: [w373] -> w310
              tunnel: [w372] -> w309
              tunnel: [w489] -> w364
              tunnel: [w496] -> w362
              tunnel: [w495] -> w342
              tunnel: [w494] -> w338
              tunnel: [w493] -> w334
              tunnel: [w490] -> w324
              tunnel: [w491] -> w322
              tunnel: [w492] -> w320
              tunnel: [w488] -> w323
              tunnel: [w487] -> w321
              tunnel: [w486] -> w319
              tunnel: w325 -> [w488]
              tunnel: w326 -> [w487]
              tunnel: w327 -> [w486]
              tunnel: w328 -> [w492]
              tunnel: w331 -> [w491]
              tunnel: w333 -> [w490]
              tunnel: w335 -> [w493]
              tunnel: w339 -> [w494]
              tunnel: w343 -> [w495]
              tunnel: w345 -> [w472]
              tunnel: w346 -> [w473]
              tunnel: w352 -> [w474]
              tunnel: w353 -> [w475]
              tunnel: w354 -> [w476]
              tunnel: w348 -> [w477]
              tunnel: w355 -> [w478]
              tunnel: w356 -> [w470]
              tunnel: w349 -> [w479]
              tunnel: w350 -> [w480]
              tunnel: w351 -> [w481]
              tunnel: w358 -> [w482]
              tunnel: w359 -> [w483]
              tunnel: w360 -> [w484]
              tunnel: w361 -> [w485]
              tunnel: w363 -> [w496]
              tunnel: w311 -> [w463]
              tunnel: w310 -> [w464]
              tunnel: w309 -> [w462]
              frame #0 {
                w416 = FALSE ("Log (T)")
                w428 = u16 0 items=["Voltage", "Current"] ("Source Mode  (0: Voltage)")
                n77 = Index Array(array=w435, index=w434) -> (element=w394:dbl)
                n78 = call "Configure Output.vi"("Source Mode  (0: Voltage)"=w428, "error in (no error)"=w436, "Compliance  Level (0.1)"="VSA_IDD(A)", "Output Level (0)"=w394, "VISA resource name"=w381) -> ("error out"=w432:errorcluster, "VISA resource name out"=w430:refnum<visa-resource-name>)  [unwired: 5 in]
                n79 = Number To Fractional String(number=w394, precision (6)=i16 2) -> (F-format string=w399:string)  [unwired: 2 in]
                n80 = call "Enable Output.vi"("error in (no error)"=w432, "Enable Output (T: Enable)"=TRUE, "VISA resource name"=w430) -> ("error out"=w433:errorcluster, "VISA resource name out"=w380:refnum<visa-resource-name>)  [unwired: 7 in]
                n81 = Concatenate Strings("VSA Sweeping Voltage ", w399) -> (w398:string)
                n82 = call "Delay T4.vi"("milliseconds to wait"=u32 50, "error in (no error)"=w433) -> ("error out"=w379:errorcluster)  [unwired: 9 in]
                n83 = local write "STATUS"(w398) -> ()
                n84 = call "Ke2000 Reading MilAmp.vi"("error in (no error)"=w379, "VISA resource name"=w411) -> ("error out"=w409:errorcluster, "uA"=w408:string, "VISA resource name out"=w395:refnum<visa-resource-name>)  [unwired: 7 in]
                n85 = for {
                  N: 16 -> [_]
                  tunnel: w408 -> [w437]
                  tunnel: [w437] -> w407 mode=indexing
                }
                "CP Current(uA)" <- w407
                n86 = call "WS1050 AD7747 READ.vi"("error in"=w409, "Log (T)"=w416, "DUT Mask Mode (All)"=WSVCAP_SHL_I2C_DUT_Mask_Mode_Enum."C1") -> ("error out"=w425:errorcluster, "AD7747 Values"=w427:string[][])  [unwired: 7 in]
                n87 = for {
                  tunnel: w427 -> [w459] mode=indexing
                  tunnel: [w457] -> w382 mode=indexing
                  tunnel: w425 -> [w458]
                  tunnel: [w458] -> w424
                  n88 = Index Array(array=w459, index=1) -> (element=w457:string)
                }
                n89 = call "WS1050 AD7747 READ.vi"("error in"=w424, "Log (T)"=w416, "DUT Mask Mode (All)"=WSVCAP_SHL_I2C_DUT_Mask_Mode_Enum."C2") -> ("error out"=w422:errorcluster, "AD7747 Values"=w421:string[][])  [unwired: 7 in]
                n90 = for {
                  tunnel: w421 -> [w455] mode=indexing
                  tunnel: [w453] -> w383 mode=indexing
                  tunnel: w422 -> [w454]
                  tunnel: [w454] -> w420
                  n91 = Index Array(array=w455, index=3) -> (element=w453:string)
                }
                n92 = call "WS1050 AD7747 READ.vi"("error in"=w420, "Log (T)"=w416, "DUT Mask Mode (All)"=WSVCAP_SHL_I2C_DUT_Mask_Mode_Enum."C3") -> ("error out"=w418:errorcluster, "AD7747 Values"=w417:string[][])  [unwired: 7 in]
                n93 = for {
                  tunnel: w417 -> [w451] mode=indexing
                  tunnel: [w449] -> w412 mode=indexing
                  tunnel: w418 -> [w450]
                  tunnel: [w450] -> w414
                  n94 = Index Array(array=w451, index=5) -> (element=w449:string)
                }
                n95 = case shown="0" w413 {
                  tunnel: w414 -> [w441 w448]
                  tunnel: [w441 w448] -> w375
                  tunnel: w412 -> [w438 w445]
                  tunnel: w383 -> [w439 w446]
                  tunnel: w382 -> [w440 w447]
                  tunnel: [w440 w447] -> w404
                  tunnel: [w439 w446] -> w405
                  tunnel: [w438 w445] -> w406
                  tunnel: [w438 w444] -> w378
                  tunnel: [w439 w443] -> w377
                  tunnel: [w440 w442] -> w376
                  frame 0 {
                    "VSA_C3_T0" <- w438
                    "VSA_C2_T0" <- w439
                    "VSA_C1_T0" <- w440
                  }
                  frame 1, Default {
                    n96 = local read "VSA_C1_T0"() -> (w442:string[])
                    n97 = local read "VSA_C2_T0"() -> (w443:string[])
                    n98 = local read "VSA_C3_T0"() -> (w444:string[])
                  }
                }
                n99 = Build Array(w382, w383, w412) -> (w385:string[][])
                n100 = Transpose 2D Array(2D array=w385) -> (transposed array=→"VSA_Value(pF)":string[][])
                n101 = call "WS1050 VSA_Delta C Calculation.vi"("error in (no error)"=w375, "VSA_T"=w404, "VSA_T0"=w376) -> ("error out"=w374:errorcluster, 2:"VSA Delta C(pF)"=w387:dbl[], 3:"VSA Delta C(pF)"=w403:string[])  [unwired: 6 in]
                n102 = call "WS1050 VSA_Delta C Calculation.vi"("error in (no error)"=w375, "VSA_T"=w405, "VSA_T0"=w377) -> ("error out"=w373:errorcluster, 2:"VSA Delta C(pF)"=w390:dbl[], 3:"VSA Delta C(pF)"=w402:string[])  [unwired: 6 in]
                n103 = call "WS1050 VSA_Delta C Calculation.vi"("error in (no error)"=w375, "VSA_T"=w406, "VSA_T0"=w378) -> ("error out"=w372:errorcluster, 2:"VSA Delta C(pF)"=w391:dbl[], 3:"VSA Delta C(pF)"=w401:string[])  [unwired: 6 in]
              }
              frame #1 {
                n104 = Concatenate Strings(w473, w472) -> (w471:string)
                n105 = Merge Errors(w463, w464, w462) -> (w461:errorcluster)
                n106 = Get Date/Time In Seconds() -> (seconds since 1Jan1904=w469:timestamp)
                n107 = call "WS1050_16 DUT VSA Save Data Ver1.0.vi"("TMN DC\\CAP Data Log File Path"=w482, "Lot#"=w481, "VSA_Delta C1(pF)"=w476, "Wafer#"=w480, "File Name"=w477, "VSA_Delta C2(pF)"=w475, "error in"=w461, "Comment"=w471, "CP Current(uA)"=w478, "VSA_IDD(A)"="NA", "VSA_C1"=w485, "VSA_C2"=w484, "SN"=w479, "VSA_C3"=w483, "Voltage(V)"=w470, "VSA_Delta C3(pF)"=w474) -> ("error out"=w489:errorcluster)  [unwired: 11 in]
                n108 = Get Date/Time String(seconds (now)=w469, want seconds? (F)=TRUE) -> (date string=→"date string":string, time string=→"Previous Time":string)  [unwired: 1 in]
              }
            }
            n109 = Increment(x=w357) -> (x+1=→"Running Loops":i32)
            n110 = Build Array (concatenate)(w334, w338) -> (w337:dbl[])
            n111 = Build Array (concatenate)(w324, w323) -> (w318:dbl[][])
            n112 = call "Delay T4.vi"("milliseconds to wait"=u32 10, "error in (no error)"=w364) -> ("error out"=w368:errorcluster)  [unwired: 9 in]
            n113 = Transpose 2D Array(2D array=w318) -> (transposed array=w317:dbl[][])
            "C1 Plot" <- w317
            n114 = Build Array (concatenate)(w322, w321) -> (w316:dbl[][])
            n115 = Transpose 2D Array(2D array=w316) -> (transposed array=w315:dbl[][])
            "C2 Plot" <- w315
            n116 = Unbundle By Name(w368) -> ("status"=w341:bool)
            n117 = local read "Abort"() -> (w340:bool)
            n118 = Build Array (concatenate)(w320, w319) -> (w314:dbl[][])
            n119 = Transpose 2D Array(2D array=w314) -> (transposed array=w313:dbl[][])
            "C3 Plot" <- w313
            n120 = Compound Arithmetic op=OR(w341, w340) -> (w367:bool)
          }
          "C1 Out" <- w243
          "Voltage Out" <- w252
          n121 = call "Convert to Dynamic Data4"("2D Array"=w243) -> ("Dynamic Data Type"=w262:dynamicdata)  [unwired: 3 in]
          n122 = call "Convert to Dynamic Data"("Array"=w252) -> ("Dynamic Data Type"=w267:dynamicdata)  [unwired: 3 in]
          n123 = call "Convert to Dynamic Data3"("Array"=w252) -> ("Dynamic Data Type"=w263:dynamicdata)  [unwired: 3 in]
          n124 = call "Convert to Dynamic Data6"("2D Array"=w259) -> ("Dynamic Data Type"=w258:dynamicdata)  [unwired: 3 in]
          n125 = call "Convert to Dynamic Data2"("Array"=w252) -> ("Dynamic Data Type"=w264:dynamicdata)  [unwired: 3 in]
          n126 = call "Convert to Dynamic Data5"("2D Array"=w261) -> ("Dynamic Data Type"=w260:dynamicdata)  [unwired: 3 in]
          n127 = call "Build XY Graph3"("error in (no error)"=w251, "Y Input"=w258, "X Input"=w263) -> ("error out"=w247:errorcluster, "XY Graph"=→"Bank 3 Graph":cluster{"Y":dbl[], "Y":dbl[]}[])  [unwired: 2 in, 5 out]
          n128 = call "Build XY Graph2"("error in (no error)"=w251, "Y Input"=w260, "X Input"=w264) -> ("error out"=w248:errorcluster, "XY Graph"=→"Bank 2 Graph":cluster{"Y":dbl[], "Y":dbl[]}[])  [unwired: 2 in, 5 out]
          n129 = call "Build XY Graph"("error in (no error)"=w251, "Y Input"=w262, "X Input"=w267) -> ("error out"=w249:errorcluster, "XY Graph"=→"Bank 1 Graph":cluster{"Y":dbl[], "Y":dbl[]}[])  [unwired: 2 in, 5 out]
          n130 = Merge Errors(w249, w248, w247) -> (w250:errorcluster)
        }
        n131 = flat-sequence {
          tunnel: w224 -> [w241]
          tunnel: [w241] -> w223
          frame #0 {
            n132 = One Button Dialog(message="Test Completed") -> ()  [unwired: 1 in, 1 out]
          }
        }
        n133 = VISA Write(VISA resource name=w225, write buffer="SOUR:FUNC VOLT;VOLT:MODE FIX;RANG 100;LEV 0.0;:SENS:FUNC \"CURR\";CURR:PROT 60E-3;RANG 100E-3;:OUTP ON", error in (no error)=w223) -> (VISA resource name out=w236:refnum<visa-resource-name>, error out=w226:errorcluster)  [unwired: 1 out]
      }
      frame True {
        w497 = FALSE
      }
    }
    n134 = Unbundle By Name(w52) -> ("status"=w69:bool)
    n135 = local write "Abort"(w49) -> ()
    n136 = local write "stop"(w50) -> ()
    n137 = Wait Until Next ms Multiple(millisecond multiple=u32 100) -> ()  [unwired: 1 out]
    n138 = Or(x=w69, y=w60) -> (x .or. y?=w68:bool)
    "STATUS" <- "Idle...." ("STATUS")
  }
  "Ke2000 Out" <- w20
  "PS1 Out" <- w19
  n139 = local write "Abort"(w3) -> ()
  n140 = local write "stop"(w3) -> ()
  n141 = case shown="True" w17 {
    tunnel: [w502 w504] -> w2
    tunnel: w11 -> [w502 w503]
    frame False {
    }
    frame True {
      n142 = flat-sequence {
        tunnel: w503 -> [w507]
        tunnel: [w506] -> w504
        frame #0 {
          n143 = local write "Online"(FALSE ("Online")) -> ()
          n144 = call "WSVCAP SHL Host TL Close.vi"("error in"=w507) -> ("error out"=w506:errorcluster)  [unwired: 14 in]
        }
      }
    }
  }
  "error out" <- w2
  n145 = VISA Write(VISA resource name=w12, write buffer="SOUR:FUNC VOLT;VOLT:MODE FIX;RANG 100;LEV 0.0;:SENS:FUNC \"CURR\";CURR:PROT 60E-3;RANG 100E-3;:OUTP OFF", error in (no error)=w11) -> (VISA resource name out=→"VISA resource name out":refnum<visa-resource-name>, error out=→"error out 2":errorcluster)  [unwired: 1 out]
